vi "TESTINGqUEUE.vi"() -> ()   [LabVIEW 2017]
uses:
  <vilib>/addons/database/Connection.llb/Conn ObjectReference.ctl
  <vilib>/addons/database/Connection.llb/DB Tools Open Connec (Path).vi
  <vilib>/addons/database/Connection.llb/Conn Execute.vi
  <vilib>/addons/database/Recordset.llb/Rec Fetch Recordset Data (R).vi
  <vilib>/addons/database/Recordset.llb/Rec Destroy - Connection.vi
  <vilib>/addons/database/NI_Database_API.lvlib
panel:
  in  "REJECTION COUNT in":i32
  in  "Station No.":string="10"
  in  "Product code":string
  out "REJ COUNT":i32
  out "error out 3":errorcluster
  out "Refnum out 2":T1
  in  "Current Shift":i32
  out "TABLE NAME":string
  out "SHIFT":i32
  out "DATE":string
  out "recordset data":variant[][](array[variant])
  out "resulting string":string
  out "REJECTION COUNT":i32
  out "MAX Rejection ID":i32
  out "error out":errorcluster
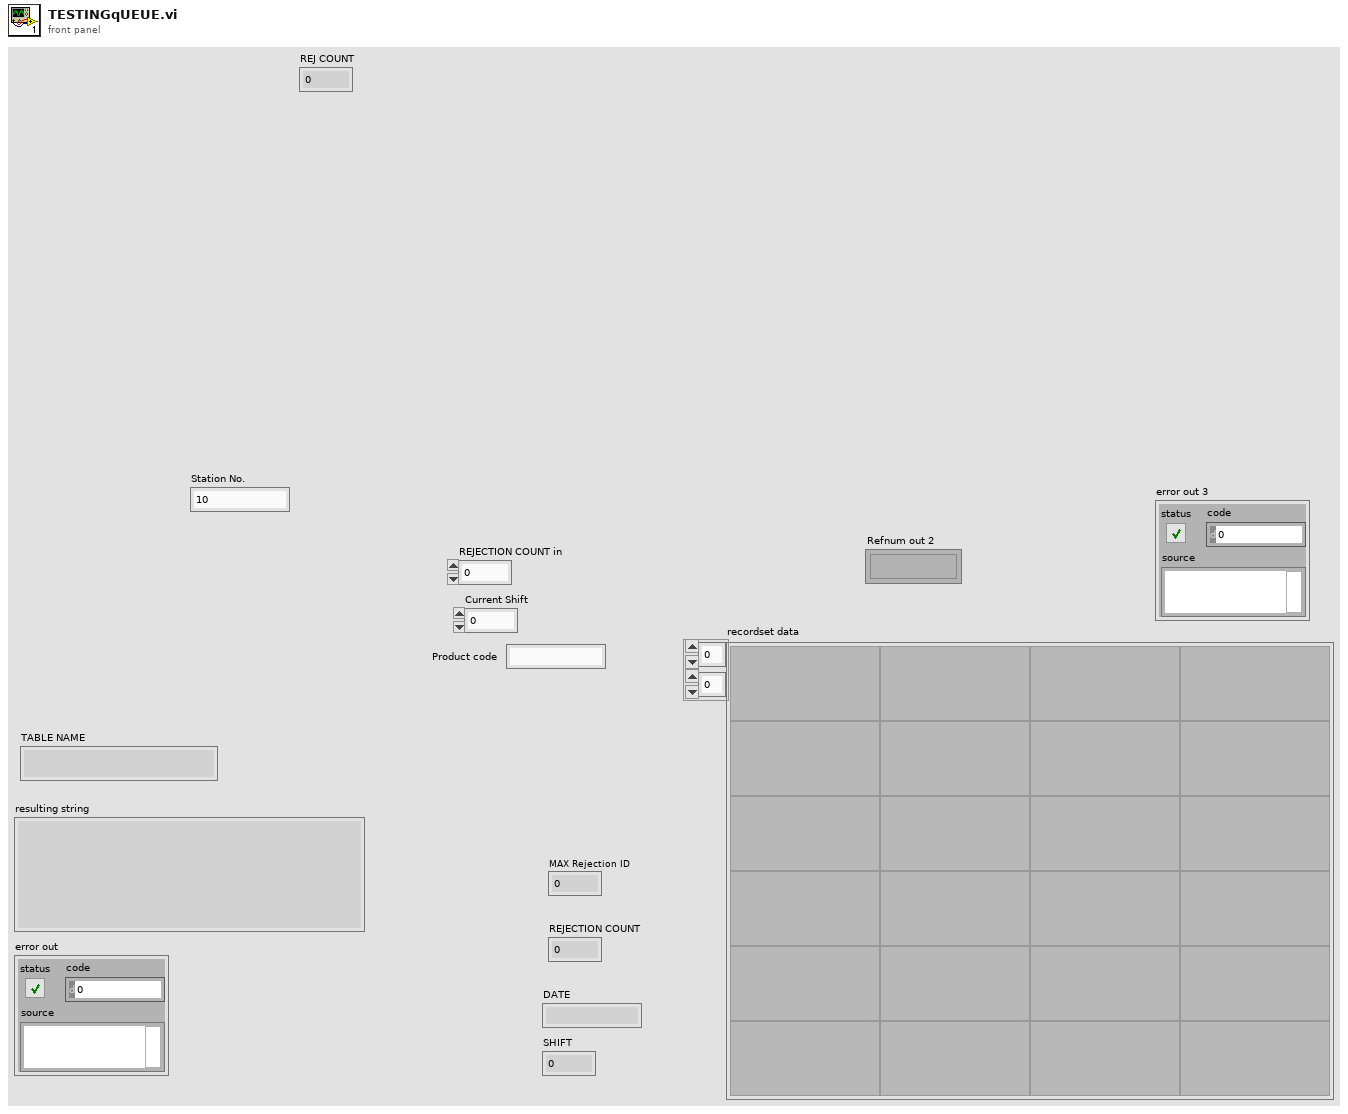
[diagram p1: front panel]
types:
  T1 = typedef "NI_Database_API.lvlib/Conn ObjectReference.ctl" = refnum<k1>
  T2 = typedef "NI_Database_API.lvlib/Rec ObjectReference.ctl" = refnum<k1>
  T3 = typedef "LVDateTimeRec.ctl" = cluster{"fractional second":dbl, "second":i32, "minute":i32, "hour":i32, "day of month":i32, "month":i32, "year":i32, "day of week":i32, "day of year":i32, "DST":i32}
  T4 = cluster{i32, "Station No.":string, "REJECTION COUNT in":i32, "Current Shift":i32, "date/time string":string, "Date String":string, "Product code":string}
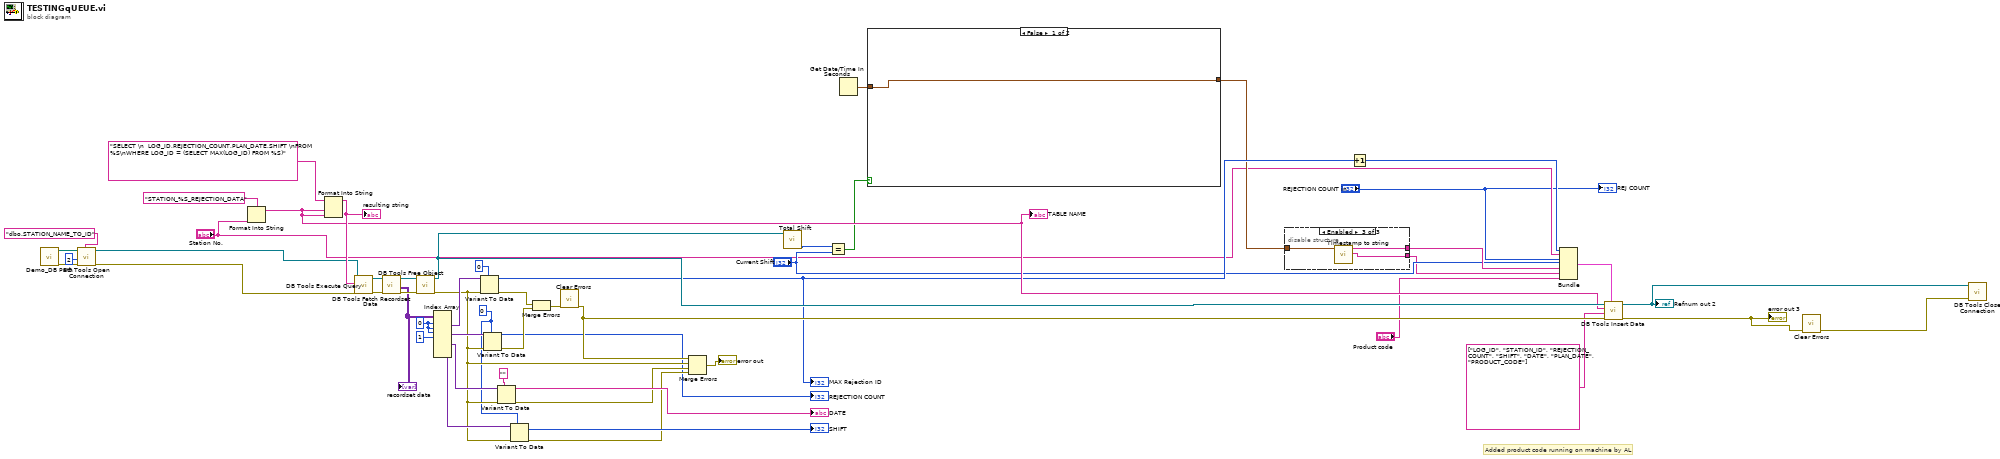
[diagram p0: block diagram]
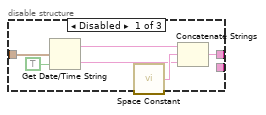
[diagram p2: hidden frame]
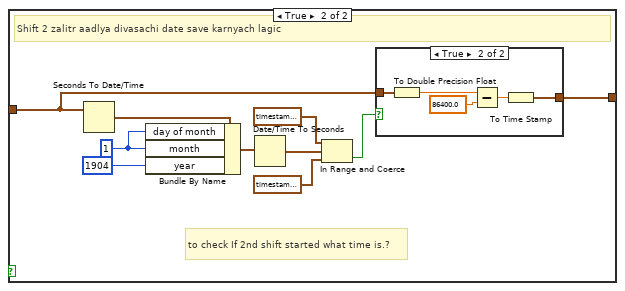
[diagram p4: hidden frame]
diagram:
  w27 = 0
  w42 = 0 ("index (row)")
  # "Added product code running on machine by AL"
  n1 = call "Demo_DB Path.vi"() -> ("error out"=w8:errorcluster, "DB Path"=w9:path)  [unwired: 10 in]
  n2 = call-poly <vilib>:"DB Tools Open Connection.vi"("userID"="dbo.STATION_NAME_TO_ID" ("table"), "error in (no error)"=w8, "connection timeout (15)"=2, "connection information"=w9) -> ("error out"=w4:errorcluster, "connection reference"=w5:T1)  [unwired: 4 in]
  n3 = Format Into String(format string="STATION_%S_REJECTION_DATA" ("SQL query"), "Station No.") -> (resulting string=w35:string)  [unwired: 2 in, 1 out]
  "TABLE NAME" <- w35
  n4 = Format Into String(format string="SELECT \n  LOG_ID,REJECTION_COUNT,PLAN_DATE,SHIFT \nFROM %S\nWHERE LOG_ID = (SELECT MAX(LOG_ID) FROM %S)" ("SQL query"), w35, w35) -> (resulting string=w46:string)  [unwired: 2 in, 1 out]
  "resulting string" <- w46
  n5 = call-poly <vilib>:"DB Tools Execute Query.vi"("error in (no error)"=w4, "SQL query"=w46, "connection reference"=w5) -> ("error out"=w50:errorcluster, "recordset reference"=w51:T2)  [unwired: 5 in]
  n6 = call-poly <vilib>:"DB Tools Fetch Recordset Data.vi"("error in (no error)"=w50, "recordset reference"=w51) -> ("error out"=w49:errorcluster, "recordset data"=w33:variant[][], "recordset reference out"=w52:T2)  [unwired: 3 in]
  "recordset data" <- w33
  n7 = call-poly <vilib>:"DB Tools Free Object.vi"("error in (no error)"=w49, "recordset reference"=w52) -> ("error out"=w28:errorcluster, "connection reference"=w36:T1)  [unwired: 8 in]
  n8 = Index Array(array=w33, index (row) #1=w42, index (col) #1=w42, index (row) #2=w42, index (col) #2=1 ("index (row)")) -> (element #1=w47:variant, element #2=w41:variant, element #3=w32:variant, element #4=w29:variant)  [unwired: 4 in]
  n9 = Variant To Data(error in=w28, type=0, Variant=w47) -> (data=w34:i32, error out=w53:errorcluster)
  "MAX Rejection ID" <- w34
  n10 = Variant To Data(error in=w28, type=w27, Variant=w41) -> (data=→"REJECTION COUNT":i32, error out=w39:errorcluster)
  n11 = Variant To Data(error in=w28, type="", Variant=w32) -> (data=→"DATE":string, error out=w25:errorcluster)
  n12 = Variant To Data(error in=w28, type=w27, Variant=w29) -> (data=→"SHIFT":i32, error out=w24:errorcluster)
  n13 = Merge Errors(w53, w39) -> (w40:errorcluster)
  n14 = call <vilib>:"Clear Errors.vi"("error in (no error)"=w40) -> ("error out"=w37:errorcluster)  [unwired: 5 in, 1 out]
  n15 = Merge Errors(w37, w28, w25, w24) -> (→"error out":errorcluster)
  n16 = call "Total Shift.vi"("connection reference"=w36) -> ("Total Shifts"=w19:i32)  [unwired: 9 in, 1 out]
  n17 = Equal?(x=w19, y="Current Shift") -> (x = y?=w20:bool)
  n18 = Get Date/Time In Seconds() -> (seconds since 1Jan1904=w18:timestamp)
  n19 = case shown="False" w20 {
    tunnel: w18 -> [w54 w55]
    tunnel: [w54 w56] -> w17
    frame False {
    }
    frame True {
      w61 = 1 ("day of month")
      # "to check If 2nd shift started what time is.?"
      # "Shift 2 zalitr aadlya divasachi date save karnyach lagic"
      n20 = Seconds To Date/Time(time stamp (now)=w55) -> (date time rec=w62:T3)  [unwired: 1 in]
      n21 = Bundle By Name(cluster=w62, "day of month"=w61, "month"=w61, "year"=1904) -> (w64:T3)
      n22 = Date/Time To Seconds(2:w64) -> (0:w60:timestamp)  [unwired: 1 in]
      n23 = In Range and Coerce(upper limit=timestamp(5399 s since 1904-01-01), x=w60, lower limit=timestamp(-19800 s since 1904-01-01)) -> (In Range?=w57:bool)  [unwired: 1 out]
      n24 = case shown="True" w57 {
        tunnel: [w65 w67] -> w56
        tunnel: w55 -> [w65 w66]
        frame False {
        }
        frame True {
          n25 = To Double Precision Float(number=w66) -> (double precision float=w70:dbl)
          n26 = Subtract(x=w70, y=86400.0) -> (x-y=w68:dbl)
          n27 = To Time Stamp(1:w68) -> (0:w67:timestamp)
        }
      }
    }
  }
  n28 = disable-structure shown="Enabled" {
    disable-tunnel: w17 -> [w76 w77 w80]
    disable-tunnel: [w72 w77 w79] -> w21
    disable-tunnel: [_ _ w78] -> w15
    frame Disabled {
      n29 = Get Date/Time String(seconds (now)=w76, want seconds? (F)=TRUE) -> (date string=w73:string, time string=w74:string)  [unwired: 1 in]
      n30 = call <vilib>:"Space Constant.vi"() -> ("String"=w75:string)
      n31 = Concatenate Strings(w73, w75, w74) -> (w72:string)
    }
    frame Disabled {
    }
    frame Enabled {
      n32 = call "Timestamp to string.vi"("time stamp"=w80) -> ("Date String"=w78:string, "date/time string"=w79:string)  [unwired: 8 in, 1 out]
    }
  }
  n33 = Increment(x=w34) -> (x+1=w22:i32)
  n34 = Bundle(w22, "Station No."="Station No.", "REJECTION COUNT in"="REJECTION COUNT in", "Current Shift"="Current Shift", "date/time string"=w21, "Date String"=w15, "Product code"="Product code") -> (w23:T4)  [unwired: 1 in]
  n35 = call <vilib>:"DB Tools Insert Data.vi"("data"=w23, "error in (no error)"=w37, "columns"=string[] ["LOG_ID", "STATION_ID", "REJECTION_COUNT", "SHIFT", "DATE", "PLAN_DATE", "PRODUCT_CODE"], "table"=w35, "connection reference"=w36) -> ("error out"=w2:errorcluster, "connection reference out"=w1:T1)  [unwired: 5 in]
  "Refnum out 2" <- w1
  "error out 3" <- w2
  n36 = call <vilib>:"Clear Errors.vi"("error in (no error)"=w2) -> ("error out"=w3:errorcluster)  [unwired: 5 in, 1 out]
  n37 = call <vilib>:"DB Tools Close Connection.vi"("error in (no error)"=w3, "connection reference"=w1) -> ()  [unwired: 5 in, 1 out]
  "REJ COUNT" <- "REJECTION COUNT in"
